vi "Get New Request ID.vi"(8 "error in":errorcluster, 11 "connection in":refnum<class "Low Level Connection.lvclass">) -> (0 "error out":errorcluster, 2 "id":u32, 3 "connection out":refnum<class "Low Level Connection.lvclass">)   [LabVIEW 2020, in "NI_SFTP.lvlib" / "Low Level Connection.lvclass"]
uses:
  <vilib>/net/SFTP/Low Level Connection/Low Level Connection.lvclass
  <vilib>/net/SFTP/Low Level Connection/Low Level Connection.lvclass/Low Level Connection.ctl
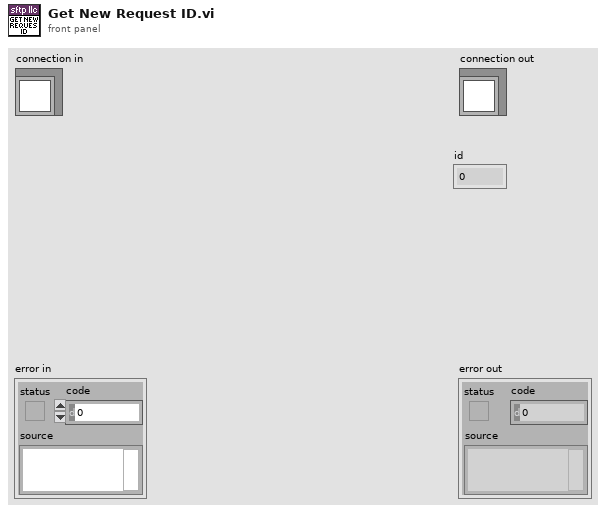
[diagram p1: front panel]
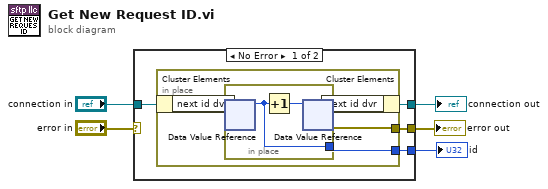
[diagram p0: block diagram]
diagram:
  n1 = case shown="No Error" "error in" {
    selector: "error in" -> [_ w17]
    tunnel: [w6 w17] -> w4
    tunnel: [w8 w16] -> w2
    tunnel: "connection in" -> [w7 w16]
    tunnel: [w9 _] -> w1
    frame No Error {
      n2 = in-place {
        in-place-border: [w12] -> w9
        in-place-border: [w10] -> w6
        n3 = in-place-cluster #1(w7) -> ("next id dvr"=w13:refnum<data-value>)
        n4 = in-place {
          in-place-border: [w14] -> w12
          n5 = in-place-dvr #2(w13) -> (w14:u32)  [unwired: 1 out]
          n6 = Increment(x=w14) -> (x+1=w15:u32)
          n7 = in-place-dvr #2(w15) -> (w11:refnum<data-value>, w10:errorcluster)
        }
        n8 = in-place-cluster #1("next id dvr"=w11) -> (w8:refnum<class "Low Level Connection.lvclass">)
      }
    }
    frame Error {
    }
  }
  "error out" <- w4
  "connection out" <- w2
  "id" <- w1
